vi "Ramp.vi"(11 "Array":dbl[][](array[numeric])) -> (0 "Result calculated from":dbl[](array[numeric]), 1 "Acceleration":dbl, 2 "Time":dbl[](array[numeric]), 3 "Distance":dbl[](array[numeric]))   [LabVIEW 2021]
uses:
  <vilib>/Analysis/NI_AALPro.lvlib
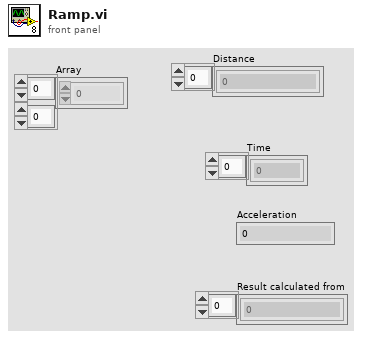
[diagram p1: front panel]
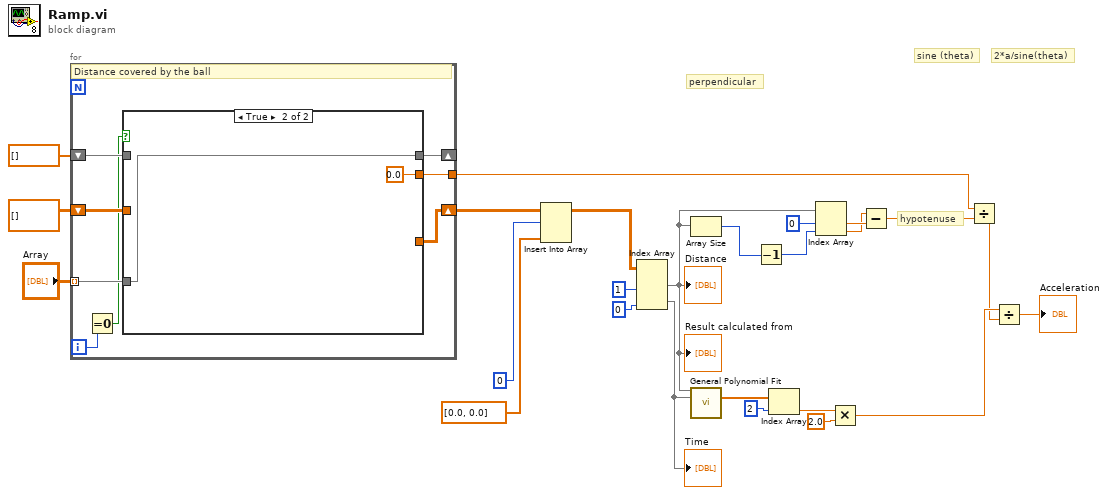
[diagram p0: block diagram]
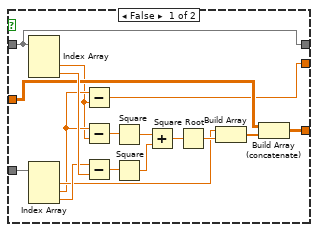
[diagram p2: hidden frame]
diagram:
  # "hypotenuse"
  # "perpendicular"
  # "2*a/sine(theta)"
  # "sine (theta)"
  n1 = for {
    tunnel: "Array" -> [w33] mode=indexing
    shift-right: [w30] -> w11
    shift-left: dbl[][] [] -> [w31]
    shift-right: [w29] -> _
    shift-left: dbl[] [] -> [w32]
    tunnel: [w28] -> w5
    i -> [w27]
    # "Distance covered by the ball"
    n2 = Equal To 0?(x=w27) -> (x = 0?=w26:bool)
    n3 = case shown="True" w26 {
      tunnel: w33 -> [w50 w52]
      tunnel: w32 -> [w38 _]
      tunnel: w31 -> [w40 _]
      tunnel: [w39 _] -> w30
      tunnel: [w38 w52] -> w29
      tunnel: [w36 0.0] -> w28
      frame False {
        n4 = Index Array(array=w38) -> (element #2=w34:dbl, element #3=w43:dbl)  [unwired: 3 in, 1 out]
        n5 = Index Array(array=w50) -> (element #1=w37:dbl, element #2=w35:dbl, element #3=w42:dbl)  [unwired: 3 in]
        n6 = Subtract(x=w35, y=w34) -> (x-y=w36:dbl)
        n7 = Subtract(x=w35, y=w34) -> (x-y=w49:dbl)
        n8 = Subtract(x=w42, y=w43) -> (x-y=w48:dbl)
        n9 = Square(x=w49) -> (x^2=w47:dbl)
        n10 = Square(x=w48) -> (x^2=w46:dbl)
        n11 = Add(x=w47, y=w46) -> (x+y=w45:dbl)
        n12 = Square Root(x=w45) -> (sqrt(x)=w44:dbl)
        n13 = Build Array(w37, w44) -> (w41:dbl[])
        n14 = Build Array (concatenate)(w40, w41) -> (w39:dbl[][])
      }
      frame True {
      }
    }
  }
  n15 = Insert Into Array(array=w11, index (row)=0, new element=dbl[] [0.0, 0.0] ("new element/subarray")) -> (w14:dbl[][])  [unwired: 1 in]
  n16 = Index Array(array=w14, index (col) #1=1 ("disabled index (row)"), index (col) #2=0 ("index (row)")) -> (element #1=w1:dbl[], element #2=w20:dbl[])  [unwired: 2 in]
  "Distance" <- w1
  "Time" <- w20
  "Result calculated from" <- w1
  n17 = Array Size(array=w1) -> (size(s)=w15:i32)
  n18 = call <vilib>:"General Polynomial Fit.vi"("Y"=w1, "X"=w20) -> ("Polynomial Coefficients"=w16:dbl[])  [unwired: 10 in, 3 out]
  n19 = Decrement(x=w15) -> (x-1=w22:i32)
  n20 = Index Array(array=w16, index=2) -> (element=w18:dbl)
  n21 = Index Array(array=w1, index #1=0 ("index"), index #2=w22) -> (element #1=w25:dbl, element #2=w24:dbl)
  n22 = Multiply(x=w18, y=2.0) -> (x*y=w3:dbl)
  n23 = Subtract(x=w24, y=w25) -> (x-y=w4:dbl)
  n24 = Divide(x=w5, y=w4) -> (x/y=w2:dbl)
  n25 = Divide(x=w3, y=w2) -> (x/y=→"Acceleration":dbl)
